vi "NMEA_ParseMessage-GPGGA.vi"(9 "Error In":errorcluster, 10 "$GPGGA-message_IN":string) -> (1 "Error Out":errorcluster, 2 "$GPGGA-message_OUT":T1={"TimeStamp"=timestamp(0 s since 1904-01-01), "Latitude"=0.0, "Latitude-Direction"=enum."", "Longitude"=1.0, "Longitude-Direction"=enum."", "GPS-Quality"=enum."GPS fix", "Number of Satellites"=0, "Horizontal Dilution of Precision"=0.0, "Altitude above Mean-Sea-Level"=0.0, "Geoidal separation"=0.0, "Time since last DGPS update"=0.0, "DGPS reference station ID"=0} {"Time since last DGPS update" format="%.02f [s]"; "Geoidal separation" format="%.02f [m]"; "Altitude above Mean-Sea-Level" format="%.02f [m]"; "Horizontal Dilution of Precision" format="%.02f [HDOP]"; "Longitude" format="%0.4f [long]"; "Latitude" format="%.04f [lat]"; "TimeStamp" format="%<%.2X>T"})   [LabVIEW 2015]
doc: "<B>GPGGA</B>\nGlobal Positioning System Fix Data"
uses:
  C:/Users/rjr5357/Downloads/NMEA_v1.0 - LV2009/NMEA_v1.0 - LV2009/NMEA_GPGGA-data.ctl
  C:/Users/rjr5357/Downloads/NMEA_v1.0 - LV2009/NMEA_v1.0 - LV2009/NMEA_LatitudeDirection.ctl
  C:/Users/rjr5357/Downloads/NMEA_v1.0 - LV2009/NMEA_v1.0 - LV2009/NMEA_LongitudeDirection.ctl
  C:/Users/rjr5357/Downloads/NMEA_v1.0 - LV2009/NMEA_v1.0 - LV2009/NMEA_GPS-Quality.ctl
  C:/Users/rjr5357/Downloads/NMEA_v1.0 - LV2009/NMEA_v1.0 - LV2009/NMEA.lvlib
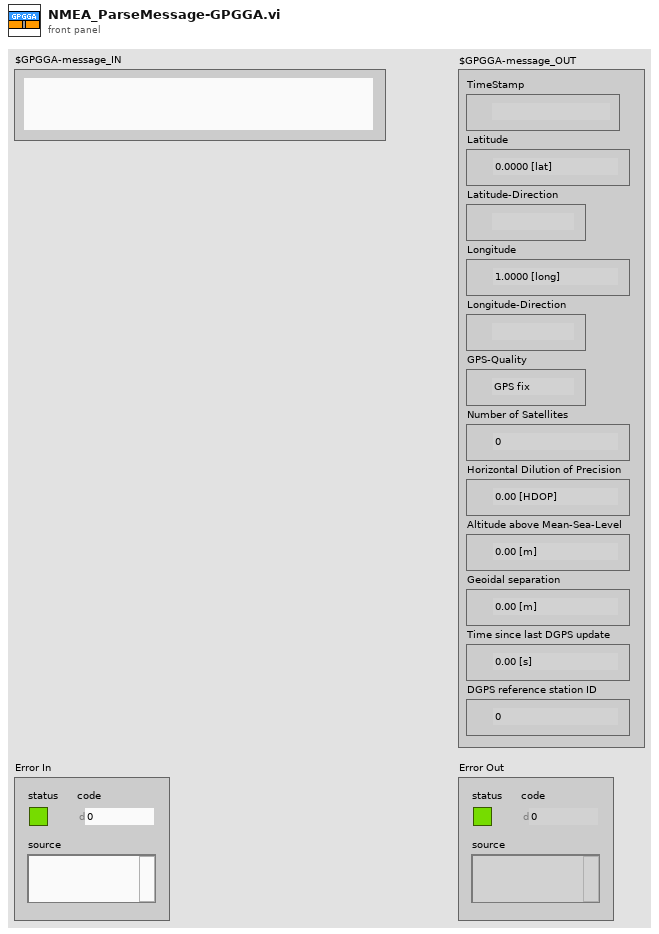
[diagram p1: front panel]
types:
  T1 = typedef "NMEA.lvlib/NMEA_GPGGA-data.ctl" = cluster{"TimeStamp":timestamp, "Latitude":dbl, "Latitude-Direction":T2, "Longitude":dbl, "Longitude-Direction":T3, "GPS-Quality":T4, "Number of Satellites":i32, "Horizontal Dilution of Precision":dbl, "Altitude above Mean-Sea-Level":dbl, "Geoidal separation":dbl, "Time since last DGPS update":dbl, "DGPS reference station ID":i32}
  T2 = typedef "NMEA.lvlib/NMEA_LatitudeDirection.ctl" = enum16{"", "North", "South"}
  T3 = typedef "NMEA.lvlib/NMEA_LongitudeDirection.ctl" = enum16{"", "East", "West"}
  T4 = typedef "NMEA.lvlib/NMEA_GPS-Quality.ctl" = enum16{"Invalid", "GPS fix", "DGPS fix"}
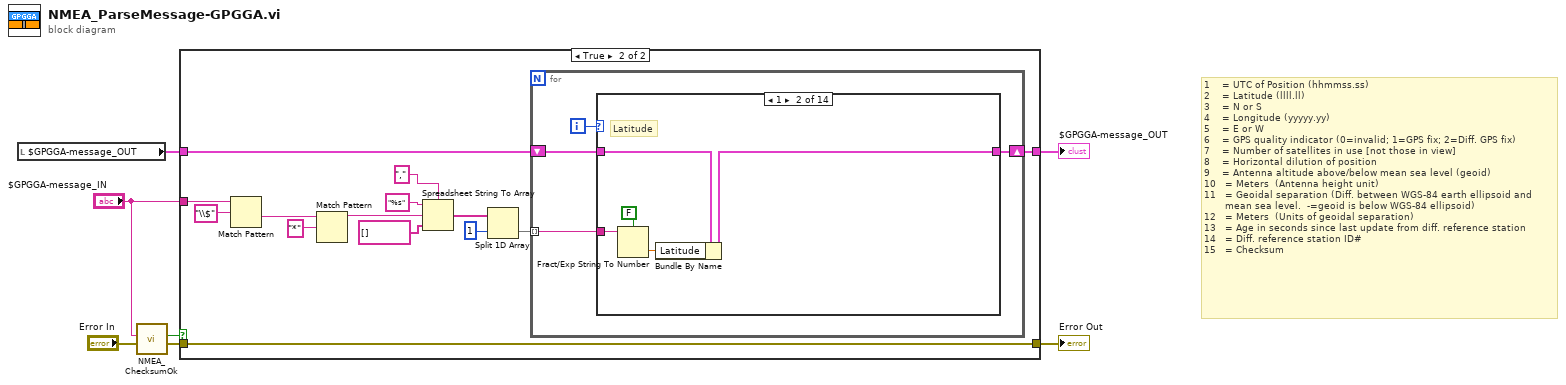
[diagram p0: block diagram]
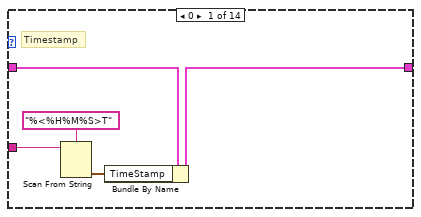
[diagram p3: hidden frame]
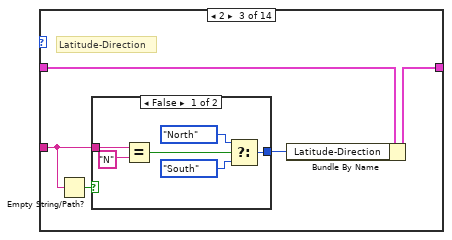
[diagram p4: hidden frame]
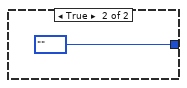
[diagram p5: hidden frame]
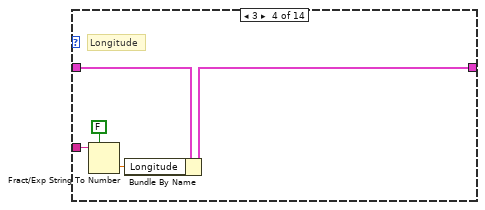
[diagram p6: hidden frame]
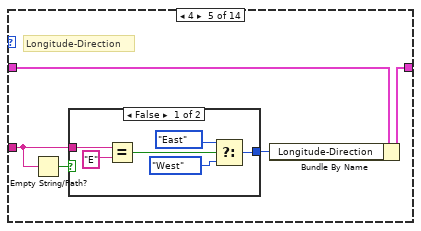
[diagram p7: hidden frame]
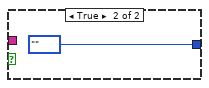
[diagram p8: hidden frame]
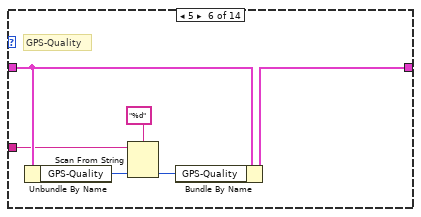
[diagram p9: hidden frame]
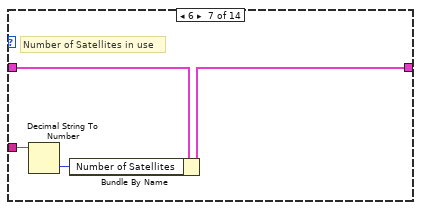
[diagram p10: hidden frame]
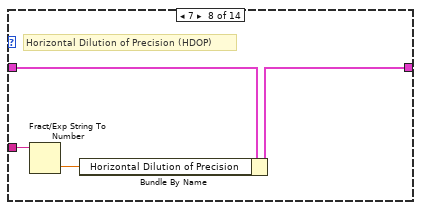
[diagram p11: hidden frame]
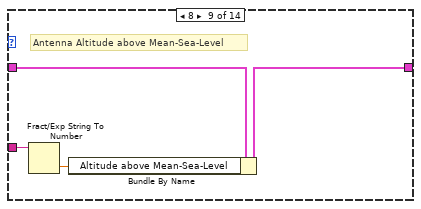
[diagram p12: hidden frame]
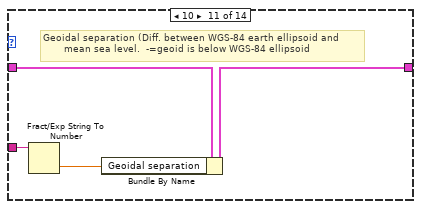
[diagram p14: hidden frame]
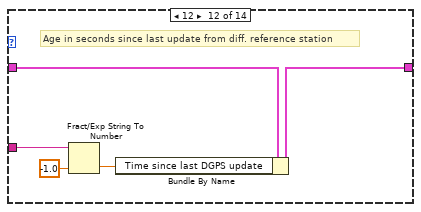
[diagram p15: hidden frame]
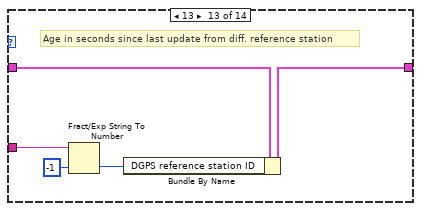
[diagram p16: hidden frame]
diagram:
  # "1    = UTC of Position (hhmmss.ss)\n2    = Latitude (llll.ll)\n3    = N or S\n4    = Longitude (yyyyy.yy)\n5    = E or W\n6    = GPS quality indicator (0=invalid; 1=GPS fix; 2=Diff. GPS fix)\n7    = Number of satellites in use [not those in view]\n8    = Horizontal dilution of position\n9    = Antenna altitude above/below mean sea level (geoid)\n10   = Meters  (Antenna height unit)\n11   = Geoidal separation (Diff. between WGS-84 earth ellipsoid and\n       mean sea level.  -=geoid is below WGS-84 ellipsoid)\n12   = Meters  (Units of geoidal separation)\n13   = Age in seconds since last update from diff. reference station\n14   = Diff. reference station ID#\n15   = Checksum"
  n1 = local read "$GPGGA-message_OUT"() -> (w7:T1)
  n2 = call "NMEA_ChecksumOk.vi"("Error In"="Error In", "Sentence"="$GPGGA-message_IN") -> ("Error Out"=w1:errorcluster, "CheckSumOk?"=w4:bool)  [unwired: 8 in]
  n3 = case shown="True" w4 {
    tunnel: w7 -> [w9 w18]
    tunnel: [w9 w17] -> w6
    tunnel: "$GPGGA-message_IN" -> [_ w15]
    tunnel: w1 -> [w8 w10]
    tunnel: [w8 w10] -> w3
    frame False {
    }
    frame True {
      n4 = Match Pattern(string=w15, regular expression="\\$") -> (after substring=w14:string)  [unwired: 1 in, 3 out]
      n5 = Match Pattern(string=w14, regular expression="*") -> (before substring=w22:string)  [unwired: 1 in, 3 out]
      n6 = Spreadsheet String To Array(delimiter (Tab)=",", format string="%s", spreadsheet string=w22, array type (2D Dbl)=string[] []) -> (array=w12:string[])
      n7 = Split 1D Array(array=w12, index=1) -> (second subarray=w13:string[])  [unwired: 1 out]
      n8 = for {
        tunnel: w13 -> [w24] mode=indexing
        shift-right: [w26] -> w17
        shift-left: w18 -> [w27]
        i -> [w25]
        n9 = case shown="1" w25 {
          tunnel: w27 -> [w32 w37 w42 w54 w59 w71 w76 w80 w84 w85 w89 w94 w99 w100]
          tunnel: [w31 w36 w41 w53 w58 w72 w75 w79 w83 w85 w88 w93 w98 w100] -> w26
          tunnel: w24 -> [w29 w35 w39 w52 w56 w68 w74 w78 w82 _ w87 w92 w97 _]
          frame 0 {
            # "Timestamp"
            n10 = Scan From String(format string="%<%H%M%S>T", input string=w29) -> (output 1=w28:timestamp)  [unwired: 3 in, 3 out]
            n11 = Bundle By Name(cluster=w32, "TimeStamp"=w28) -> (w31:T1)
          }
          frame 1 {
            # "Latitude"
            n12 = Fract/Exp String To Number(use system decimal point (T)=FALSE, string=w35) -> (number=w34:dbl)  [unwired: 2 in, 1 out]
            n13 = Bundle By Name(cluster=w37, "Latitude"=w34) -> (w36:T1)
          }
          frame 2 {
            # "Latitude-Direction"
            n14 = Empty String/Path?(string/path=w39) -> (empty?=w38:bool)
            n15 = case shown="False" w38 {
              tunnel: [w45 NMEA_LatitudeDirection."" ("f")] -> w40
              tunnel: w39 -> [w43 _]
              frame False {
                n16 = Equal?(x=w43, y="N") -> (x = y?=w47:bool)
                n17 = Select(t=NMEA_LatitudeDirection."North" ("Latitude-Direction"), s=w47, f=NMEA_LatitudeDirection."South") -> (s? t:f=w45:T2)
              }
              frame True {
              }
            }
            n18 = Bundle By Name(cluster=w42, "Latitude-Direction"=w40) -> (w41:T1)
          }
          frame 3 {
            # "Longitude"
            n19 = Fract/Exp String To Number(use system decimal point (T)=FALSE, string=w52) -> (number=w51:dbl)  [unwired: 2 in, 1 out]
            n20 = Bundle By Name(cluster=w54, "Longitude"=w51) -> (w53:T1)
          }
          frame 4 {
            # "Longitude-Direction"
            n21 = Empty String/Path?(string/path=w56) -> (empty?=w55:bool)
            n22 = case shown="False" w55 {
              tunnel: w56 -> [w65 _]
              tunnel: [w61 NMEA_LongitudeDirection."" ("f")] -> w57
              frame False {
                n23 = Equal?(x=w65, y="E") -> (x = y?=w63:bool)
                n24 = Select(t=NMEA_LongitudeDirection."East" ("Longitude-Direction"), s=w63, f=NMEA_LongitudeDirection."West") -> (s? t:f=w61:T3)
              }
              frame True {
              }
            }
            n25 = Bundle By Name(cluster=w59, "Longitude-Direction"=w57) -> (w58:T1)
          }
          frame 5 {
            # "GPS-Quality"
            n26 = Unbundle By Name(w71) -> ("GPS-Quality"=w70:T4)
            n27 = Scan From String(format string="%d", input string=w68, default 1=w70) -> (output 1=w69:T4)  [unwired: 2 in, 3 out]
            n28 = Bundle By Name(cluster=w71, "GPS-Quality"=w69) -> (w72:T1)
          }
          frame 6 {
            # "Number of Satellites in use"
            n29 = Decimal String To Number(string=w74) -> (number=w73:i32)  [unwired: 2 in, 1 out]
            n30 = Bundle By Name(cluster=w76, "Number of Satellites"=w73) -> (w75:T1)
          }
          frame 7 {
            # "Horizontal Dilution of Precision (HDOP)"
            n31 = Fract/Exp String To Number(string=w78) -> (number=w77:dbl)  [unwired: 3 in, 1 out]
            n32 = Bundle By Name(cluster=w80, "Horizontal Dilution of Precision"=w77) -> (w79:T1)
          }
          frame 8 {
            # "Antenna Altitude above Mean-Sea-Level"
            n33 = Fract/Exp String To Number(string=w82) -> (number=w81:dbl)  [unwired: 3 in, 1 out]
            n34 = Bundle By Name(cluster=w84, "Altitude above Mean-Sea-Level"=w81) -> (w83:T1)
          }
          frame 9, 11 {
            # "[9] - Meters (antenna height unit)\n[11] - Meters (units of geoidal separation)"
          }
          frame 10 {
            # "Geoidal separation (Diff. between WGS-84 earth ellipsoid and\n       mean sea level.  -=geoid is below WGS-84 ellipsoid"
            n35 = Fract/Exp String To Number(string=w87) -> (number=w86:dbl)  [unwired: 3 in, 1 out]
            n36 = Bundle By Name(cluster=w89, "Geoidal separation"=w86) -> (w88:T1)
          }
          frame 12 {
            # "Age in seconds since last update from diff. reference station"
            n37 = Fract/Exp String To Number(string=w92, default (0 dbl)=-1.0 ("default (0 DBL)")) -> (number=w91:dbl)  [unwired: 2 in, 1 out]
            n38 = Bundle By Name(cluster=w94, "Time since last DGPS update"=w91) -> (w93:T1)
          }
          frame 13 {
            # "Age in seconds since last update from diff. reference station"
            n39 = Fract/Exp String To Number(string=w97, default (0 dbl)=-1 ("DGPS reference station ID")) -> (number=w96:i32)  [unwired: 2 in, 1 out]
            n40 = Bundle By Name(cluster=w99, "DGPS reference station ID"=w96) -> (w98:T1)
          }
          frame Default {
          }
        }
      }
    }
  }
  "$GPGGA-message_OUT" <- w6
  "Error Out" <- w3
